vi "Drop Instrument Msg.vi"(11 "Instrument Msg in":refnum<class "Instrument Msg.lvclass">) -> ()   [LabVIEW 2020, in "Instrument Handler.lvlib" / "Instrument Msg.lvclass"]
doc: "Drop the Instrument Msg."
uses:
  Instrument Msg.lvclass
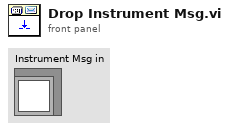
[diagram p1: front panel]
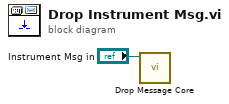
[diagram p0: block diagram]
diagram:
  n1 = call-dynamic "Drop Message Core.vi"("Response Msg in"="Instrument Msg in") -> ()  [unwired: 11 in]
